vi "Email fichier.vi"(1 "attachments":path[](array[path]), 2 "nb idice nv3":dbl, 3 "moyenne":dbl, 4 "Temp exp":dbl) -> ()   [LabVIEW 2022 SP3]
uses:
  <vilib>/smtpClient/Set Message Text.vi
  <vilib>/smtpClient/LabVIEWSMTPClient.lvlib
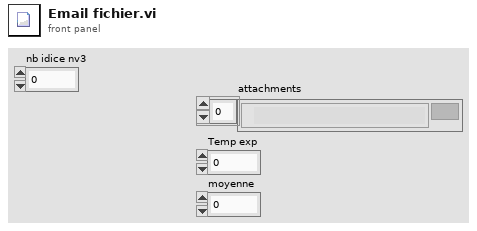
[diagram p1: front panel]
types:
  T1 = typedef "LabVIEWSMTPClient.lvlib/SmtpClientHandle.ctl" = refnum<k1>
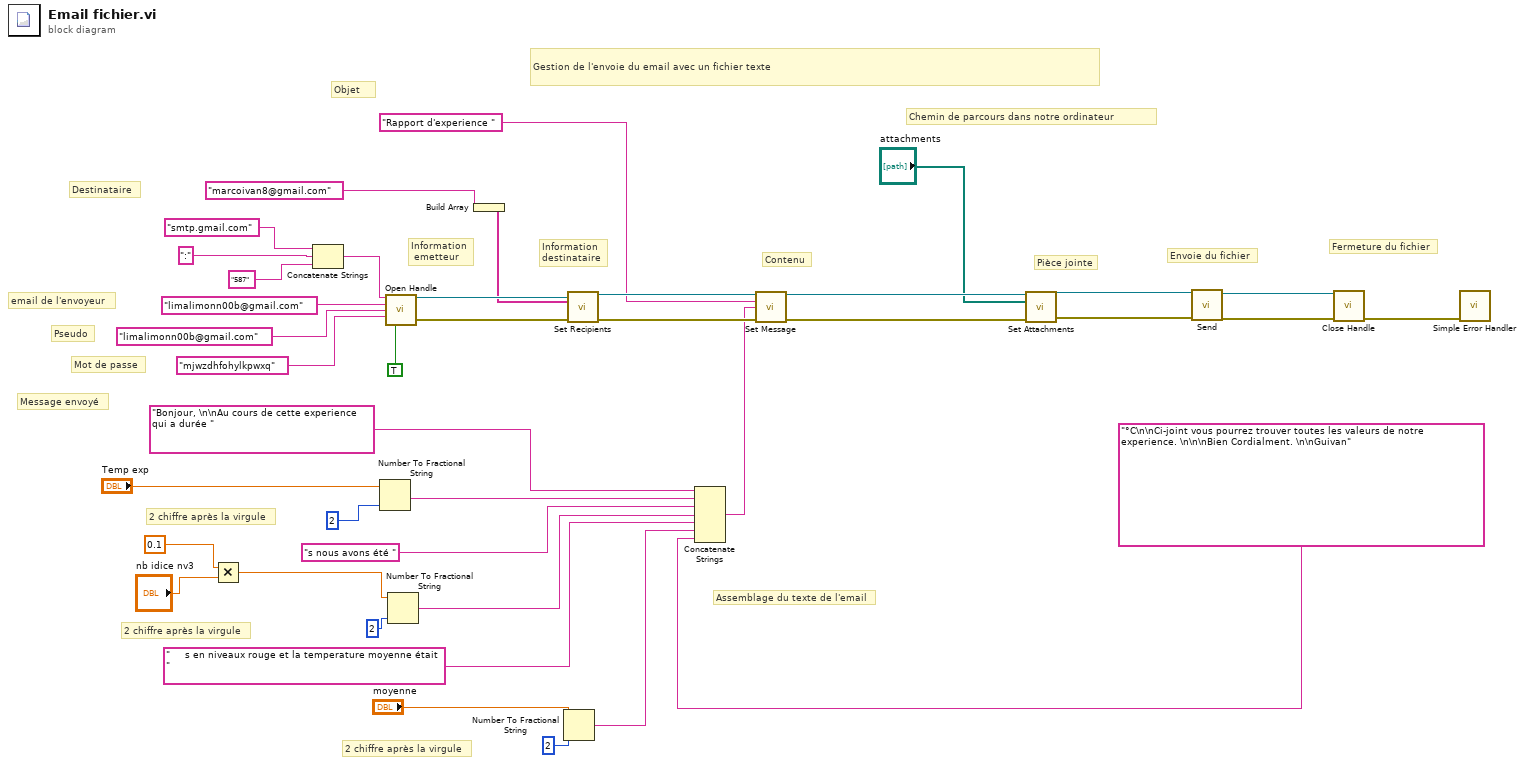
[diagram p0: block diagram]
diagram:
  # "Gestion de l'envoie du email avec un fichier texte"
  # "Information\n emetteur"
  # "Information \ndestinataire"
  # "Contenu"
  # "Envoie du fichier"
  # "Pièce jointe"
  # "Fermeture du fichier"
  # "Assemblage du texte de l'email"
  # "2 chiffre après la virgule"
  # "2 chiffre après la virgule"
  # "Message envoyé"
  # "Chemin de parcours dans notre ordinateur"
  # "2 chiffre après la virgule"
  # "Mot de passe"
  # "Pseudo"
  # "email de l'envoyeur"
  # "Destinataire"
  # "Objet"
  n1 = Multiply(x=0.1, y="nb idice nv3") -> (x*y=w1:dbl)
  n2 = Concatenate Strings("smtp.gmail.com" ("string"), ":" ("string"), "587" ("string")) -> (w23:string)
  n3 = Number To Fractional String(number="Temp exp", precision (6)=i16 2) -> (F-format string=w14:string)  [unwired: 2 in]
  n4 = call <vilib>:"Open Handle.vi"("server address"=w23, "from"="limalimonn00b@gmail.com", "username"="limalimonn00b@gmail.com", "password"="mjwzdhfohylkpwxq", "use TLS (false)"=TRUE) -> ("handle out"=w39:T1, "error out"=w29:errorcluster)  [unwired: 9 in]
  n5 = Number To Fractional String(number=w1, precision (6)=i16 2) -> (F-format string=w9:string)  [unwired: 2 in]
  n6 = Build Array("marcoivan8@gmail.com") -> (w10:string[])
  n7 = Number To Fractional String(number="moyenne", precision (6)=i16 2) -> (F-format string=w5:string)  [unwired: 2 in]
  n8 = call <vilib>:"Set Recipients.vi"("handle in"=w39, "to"=w10, "error in (no error)"=w29) -> ("handle out"=w38:T1, "error out"=w30:errorcluster)  [unwired: 11 in]
  n9 = Concatenate Strings("Bonjour, \n\nAu cours de cette experience qui a durée " ("string"), w14, "s nous avons été " ("string"), w9, "     s en niveaux rouge et la temperature moyenne était  " ("string"), w5, "°C\n\nCi-joint vous pourrez trouver toutes les valeurs de notre experience. \n\n\nBien Cordialment. \n\nGuivan" ("string")) -> (w25:string)
  n10 = call-poly <vilib>:"Set Message.vi"("handle in"=w38, "subject"="Rapport d'experience ", "plain text message"=w25, "error in (no error)"=w30) -> ("handle out"=w37:T1, "error out"=w31:errorcluster)  [unwired: 10 in]
  n11 = call <vilib>:"Set Attachments.vi"("handle in"=w37, "attachments"="attachments", "error in (no error)"=w31) -> ("handle out"=w36:T1, "error out"=w32:errorcluster)  [unwired: 11 in]
  n12 = call <vilib>:"Send.vi"("handle in"=w36, "error in (no error)"=w32) -> ("handle out"=w35:T1, "error out"=w33:errorcluster)  [unwired: 11 in, 1 out]
  n13 = call <vilib>:"Close Handle.vi"("handle in"=w35, "error in (no error)"=w33) -> ("error out"=w34:errorcluster)  [unwired: 12 in, 1 out]
  n14 = call <vilib>:"Simple Error Handler.vi"("error in (no error)"=w34) -> ()  [unwired: 4 in, 5 out]
